vi "Write APU 1.3 Speed.vi"(8 "error in (no error)":errorcluster, 10 "speed (RPM)":dbl, 11 "APU in":refnum<class "APU.lvclass">) -> (0 "error out":errorcluster, 3 "APU out":refnum<class "APU.lvclass">)   [LabVIEW 2013, in "APU.lvclass"]
uses:
  APU.lvclass
  Engine Simulation IP.lvclass/Engine Simulation IP.ctl
  APU.lvclass/APU.ctl
  <vilib>/rvi/interface/common/niFpgaWaitOnOcc.vi
  <vilib>/Utility/error.llb/Error Cluster From Error Code.vi
  <vilib>/rvi/errors/niLvFpgaAdjustHostInterfaceError.vi
  <vilib>/rvi/interface/nirviReadWriteControl/nirviReadWriteControl.xnode
  <vilib>/rvi/interface/Simulation/niFpgaSimulationCallBeginRW.vi
  NiFpgaLv.dll
  Engine Simulation IP.lvclass
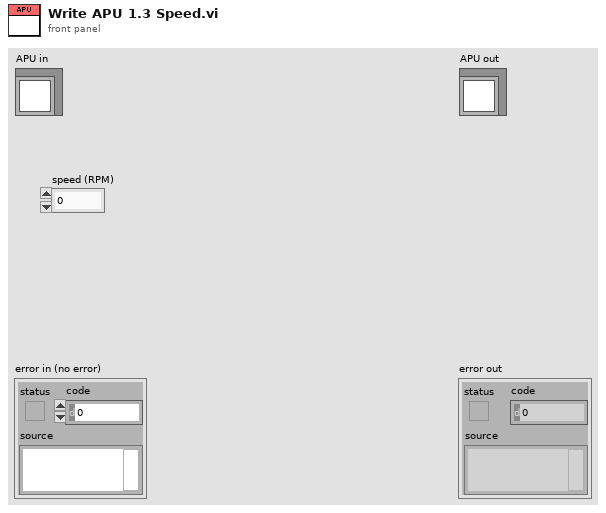
[diagram p1: front panel]
types:
  T1 = cluster{"desired speed":fxp<+/-,23,2>, "reset":bool}
  T2 = typedef "Engine Simulation Session.lvclass/Bitfile Major Version.ctl" = enum16{"1.0", "1.1", "1.2", "1.3"}
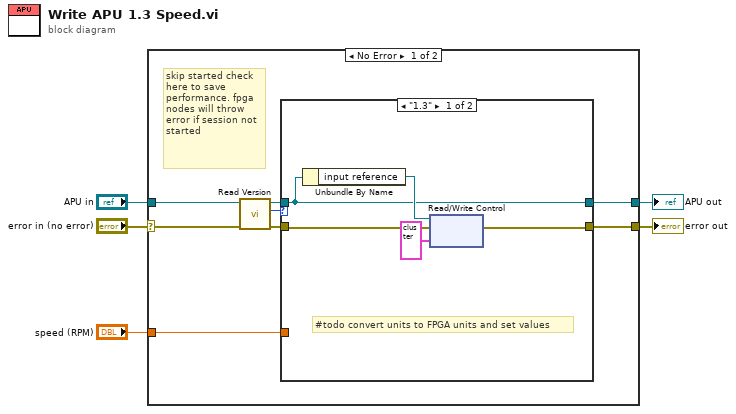
[diagram p0: block diagram]
diagram:
  n1 = case shown="No Error" "error in (no error)" {
    selector: "error in (no error)" -> [w10 w22]
    tunnel: [w13 w22] -> w4
    tunnel: [w12 w21] -> w2
    tunnel: "APU in" -> [w9 w21]
    tunnel: "speed (RPM)" -> [w11 _]
    frame No Error {
      # "skip started check here to save performance. fpga nodes will throw error if session not started"
      n2 = call "Read Version.vi"("error in (no error)"=w10, "Engine Simulation IP in"=w9) -> ("error out"=w8:errorcluster, "version"=w7:T2, "Engine Simulation IP out"=w6:refnum<class "APU.lvclass">)  [unwired: 7 in]
      n3 = case shown="\"1.3\"" w7 {
        tunnel: [w18 w20] -> w13
        tunnel: w8 -> [w16 w20]
        tunnel: w6 -> [w14 w19]
        tunnel: [w14 w19] -> w12
        tunnel: w11 -> [_ _]
        frame "1.3" {
          # "#todo convert units to FPGA units and set values"
          n4 = Unbundle By Name(w14) -> ("input reference"=w15:refnum<k20>)
          n5 = xnode "Read/Write Control"("FPGA VI Reference In"=w15, "error in"=w16, "Value"=T1 {"desired speed"=0.0, "reset"=FALSE}) -> ("error out"=w18:errorcluster)  [unwired: 1 out]
        }
        frame Default {
          # "#todo throw wrong version error"
        }
      }
    }
    frame Error {
    }
  }
  "error out" <- w4
  "APU out" <- w2
